vi "FPGAcode4_Test.vi"() -> ()   [LabVIEW 2015]
uses:
  Limits_In.ctl
  Discard_Points.ctl
  Filter_Cluster.ctl
  <vilib>/Platform/TimedLoop/XDataNode/timing_clust.ctl
  <vilib>/Platform/TimedLoop/XDataNode/nitl_modes.ctl
  <vilib>/Platform/TimedLoop/XDataNode/wakeup.ctl
  Detector_Cluster.ctl
  Correlations.ctl
  <vilib>/rvi/Emulation/niFpgaGetClockAttributes.vi
  <vilib>/rvi/Emulation/niFpgaSctlEmulationGetInTimedLoop.vi
  <vilib>/rvi/Emulation/niFpgaEmulationReportErrorSimple.vi
  <vilib>/rvi/Emulation/niFpgaProcessEmulError.vi
  <vilib>/rvi/eio/common/nirviEmuTemplateMethod_errors.vi
  <vilib>/rvi/Emulation/niFpgaCriticalErrorInLSC.vi
  <vilib>/eio/EIONode/EIONode.xnode
  <vilib>/Platform/TimedLoop/XDataNode/XDataNode.xnode
  <vilib>/Platform/TimedLoop/XDataNode/XDNodeRunTimeDep.lvlib
panel:
  in  "User Trigger?":bool
  out "Charge":T1
  out "Mass":T2
  out "Velocity Count":T3
  in  "User Trigger Distance":fxp<+/-,34,18> format="%.3g"
  out "User Trigger":bool
  out "Particles Discarded":i16
  out "All Discard Points":T4
  in  "Boxcar 3 Size Factor":fxp<+/-,32,16>=0.1999969482421875 format="%.2g"
  in  "Charge Error Factor":fxp<+/-,32,16>=1.100006103515625 format="%.2g"
  in  "Max Correlation Factor":fxp<+,32,4>=0.25 format="%.3g"
  in  "Threshold Factor":fxp<+/-,32,16>=1.0 format="%.2g"
  out "DCS 2":bool
  out "Detectors":cluster{"Det 1":i16, "Det 3":i16}
  out "DCS 1":bool
  in  "Limits":T6
  in  "Calibrate":bool=TRUE
  in  "Armed":bool
  out "Plates":bool
  in  "One Shot":bool
  # "These factors above are in the front\npanel so it is possible to experiment\nwith many different configurations\nof the FPGA on the fly. One can even\nchange the relative size of one filter."
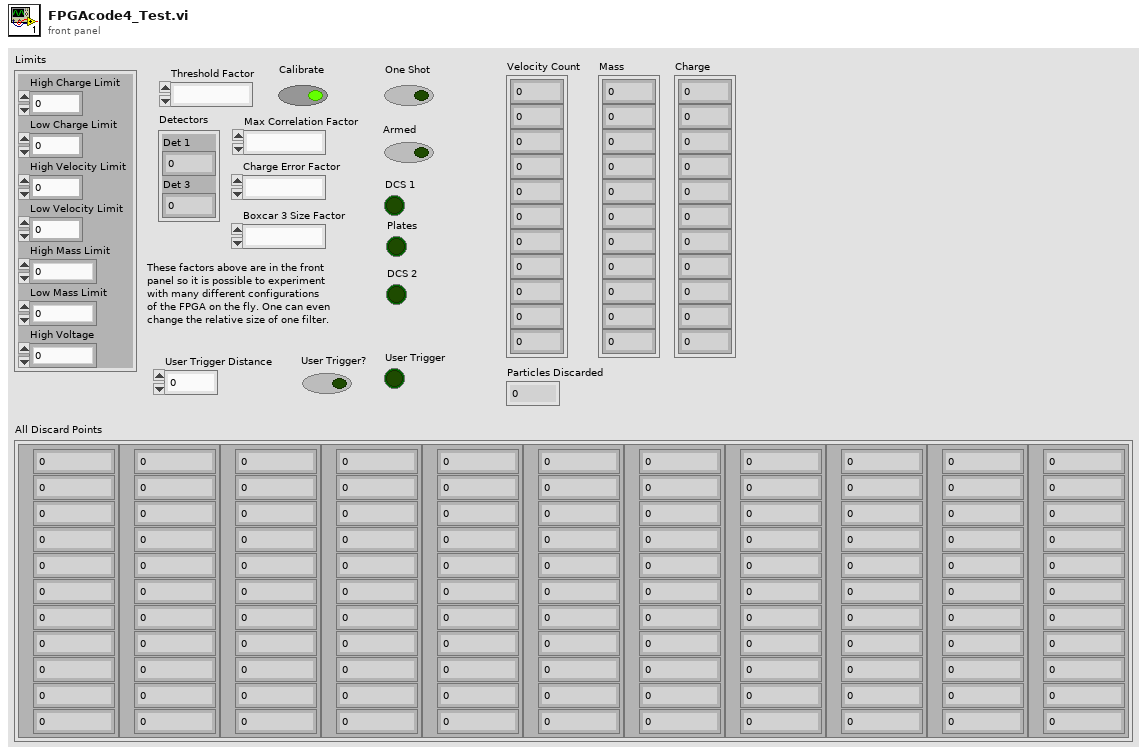
[diagram p1: front panel]
types:
  T1 = cluster{"[0]":fxp<+/-,64,-10>, "[1]":fxp<+/-,64,-10>, "[2]":fxp<+/-,64,-10>, "[3]":fxp<+/-,64,-10>, "[4]":fxp<+/-,64,-10>, "[5]":fxp<+/-,64,-10>, "[6]":fxp<+/-,64,-10>, "[7]":fxp<+/-,64,-10>, "[8]":fxp<+/-,64,-10>, "[9]":fxp<+/-,64,-10>, "[10]":fxp<+/-,64,-10>}
  T2 = cluster{"[0]":fxp<+/-,64,-2>, "[1]":fxp<+/-,64,-2>, "[2]":fxp<+/-,64,-2>, "[3]":fxp<+/-,64,-2>, "[4]":fxp<+/-,64,-2>, "[5]":fxp<+/-,64,-2>, "[6]":fxp<+/-,64,-2>, "[7]":fxp<+/-,64,-2>, "[8]":fxp<+/-,64,-2>, "[9]":fxp<+/-,64,-2>, "[10]":fxp<+/-,64,-2>}
  T3 = cluster{"[0]":i32, "[1]":i32, "[2]":i32, "[3]":i32, "[4]":i32, "[5]":i32, "[6]":i32, "[7]":i32, "[8]":i32, "[9]":i32, "[10]":i32}
  T4 = typedef "Discard_Points.ctl" = cluster{"Discard Points 1":T5, "Discard Points 2":T5, "Discard Points 3":T5, "Discard Points 4":T5, "Discard Points 5":T5, "Discard Points 6":T5, "Discard Points 7":T5, "Discard Points 8":T5, "Discard Points 9":T5, "Discard Points 10":T5, "Discard Points 11":T5}
  T5 = typedef "Filter_Cluster.ctl" = cluster{"1":i32, "2":i32, "3":i32, "4":i32, "5":i32, "6":i32, "7":i32, "8":i32, "9":i32, "10":i32, "11":i32}
  T6 = typedef "Limits_In.ctl" = cluster{"High Charge Limit":fxp<+,32,-41>, "Low Charge Limit":fxp<+,32,-41>, "High Velocity Limit":fxp<+,18,18>, "Low Velocity Limit":fxp<+,18,18>, "High Mass Limit":fxp<+/-,33,-35>, "Low Mass Limit":fxp<+/-,33,-35>, "High Voltage":fxp<+,16,22>}
  T7 = typedef "Detector_Cluster.ctl" = cluster{"Det 1":i32, "Det 2":i32}
  T8 = cluster{"Filter 1":T7, "Filter 2":T7, "Filter 3":T7, "Filter 4":T7}
  T9 = cluster{"Distance to PSU":fxp<+/-,32,5>, "Distance to end of PSU":fxp<+/-,32,5>, "Distance to DCS 2":fxp<+/-,32,5>, "Distance to DCS 1":fxp<+/-,32,5>, "Distance to front of LEIL Chamber":fxp<+/-,32,5>}
  T10 = cluster{"Detector Max Speed Count":i32, "Detector Min Speed Count":i32, "Gap Max Speed Count":i32, "Gap Min Speed Count":i32}
  T11 = cluster{"Distance to PSU":fxp<+/-,64,22>, "Distance to end of PSU":fxp<+/-,64,22>, "Distance to DCS 2":fxp<+/-,64,22>, "Distance to DCS 1":fxp<+/-,64,22>, "Distance to front of LEIL Chamber":fxp<+/-,64,22>}
  T12 = typedef "XDNodeRunTimeDep.lvlib/timing_clust.ctl" = cluster{"Expected End [f-1]":u64, "Actual End [f-1]":u64, "Finished Late? [f-1]":bool, "Expected End [i-1]":u64, "Actual End [i-1]":u64, "Finished Late? [i-1]":bool, "Expected Start [i]":u64, "Actual Start [i]":u64, "Expected Start [f]":u64, "Actual Start [f]":u64, "Source Name":string, "Structure Name":string, "Period":i64, "Deadline":i64, "Offset":i64, "Start":i64, "Priority":i32, "Timeout":i32, "Mode":T13, "Wakeup Reason":T14, "Error":errorcluster, "Source Type":string, "Secondary Source Type":string, "Global End Time":u64, "Global Start Time":u64, "Frame Duration":u64, "Iteration Duration":u64, "Assigned CPU":i32, "I/O Scan Engine Mode":u32}
  T13 = typedef "XDNodeRunTimeDep.lvlib/nitl_modes.ctl" = enum32{"No Change", "Process missed periods, maintain original phase", "Discard missed periods, maintain original phase", "Process missed periods, ignore original phase", "Discard missed periods, ignore original phase"}
  T14 = typedef "XDNodeRunTimeDep.lvlib/wakeup.ctl" = enum32{"Normal", "Aborted", "Asynchronous wakeup", "Timing source error", "Timed loop error", "Timeout"}
  T15 = cluster{"Filter 1":T7, "Filter 2":T7, "Filter 3":T7, "Filter 4":T7}[]
  T16 = cluster{"Distance to PSU":i32, "Distance to end of PSU":i32, "Distance to DCS 2":i32, "Distance to DCS 1":i32, "Distance to front of LEIL Chamber":i32}
  T17 = cluster{"First Detector Count":i32, "Detector Gap Count":i32, "Second Detector Count":i32, "Second Detector Final Count":i32}
  T18 = typedef "Correlations.ctl" = cluster{"First Correlation":i32, "Latest Correlation":i32}
  T19 = cluster{"Detectors":cluster{"Det 1":i16, "Det 3":i16}, cluster{"Det 1":i16, "Det 2":i16}, cluster{"Det 1":i16, "Det 2":i16}, cluster{"Det 1":i16, "Det 2":i16}}
  T20 = cluster{cluster{"Det 1":i16, "Det 2":i16}, cluster{"Det 1":i16, "Det 2":i16}, cluster{"Det 1":i16, "Det 2":i16}, cluster{"Det 1":i16, "Det 2":i16}}
  T21 = cluster{"[0]":u8, "[1]":u8, "[2]":u8, "[3]":u8, "[4]":u8, "[5]":u8, "[6]":u8, "[7]":u8, "[8]":u8, "[9]":u8, "[10]":u8}
  T22 = cluster{"All Discard Points[0]":T5, "All Discard Points[1]":T5, "All Discard Points[2]":T5, "All Discard Points[3]":T5, "All Discard Points[4]":T5, "All Discard Points[5]":T5, "All Discard Points[6]":T5, "All Discard Points[7]":T5, "All Discard Points[8]":T5, "All Discard Points[9]":T5, "All Discard Points[10]":T5}
  T23 = cluster{i32[], fxp<+/-,64,-2>[], fxp<+/-,64,-10>[]}
  T24 = cluster{"IO Module\\AI 0":i16, "IO Module\\AI 1":i16}
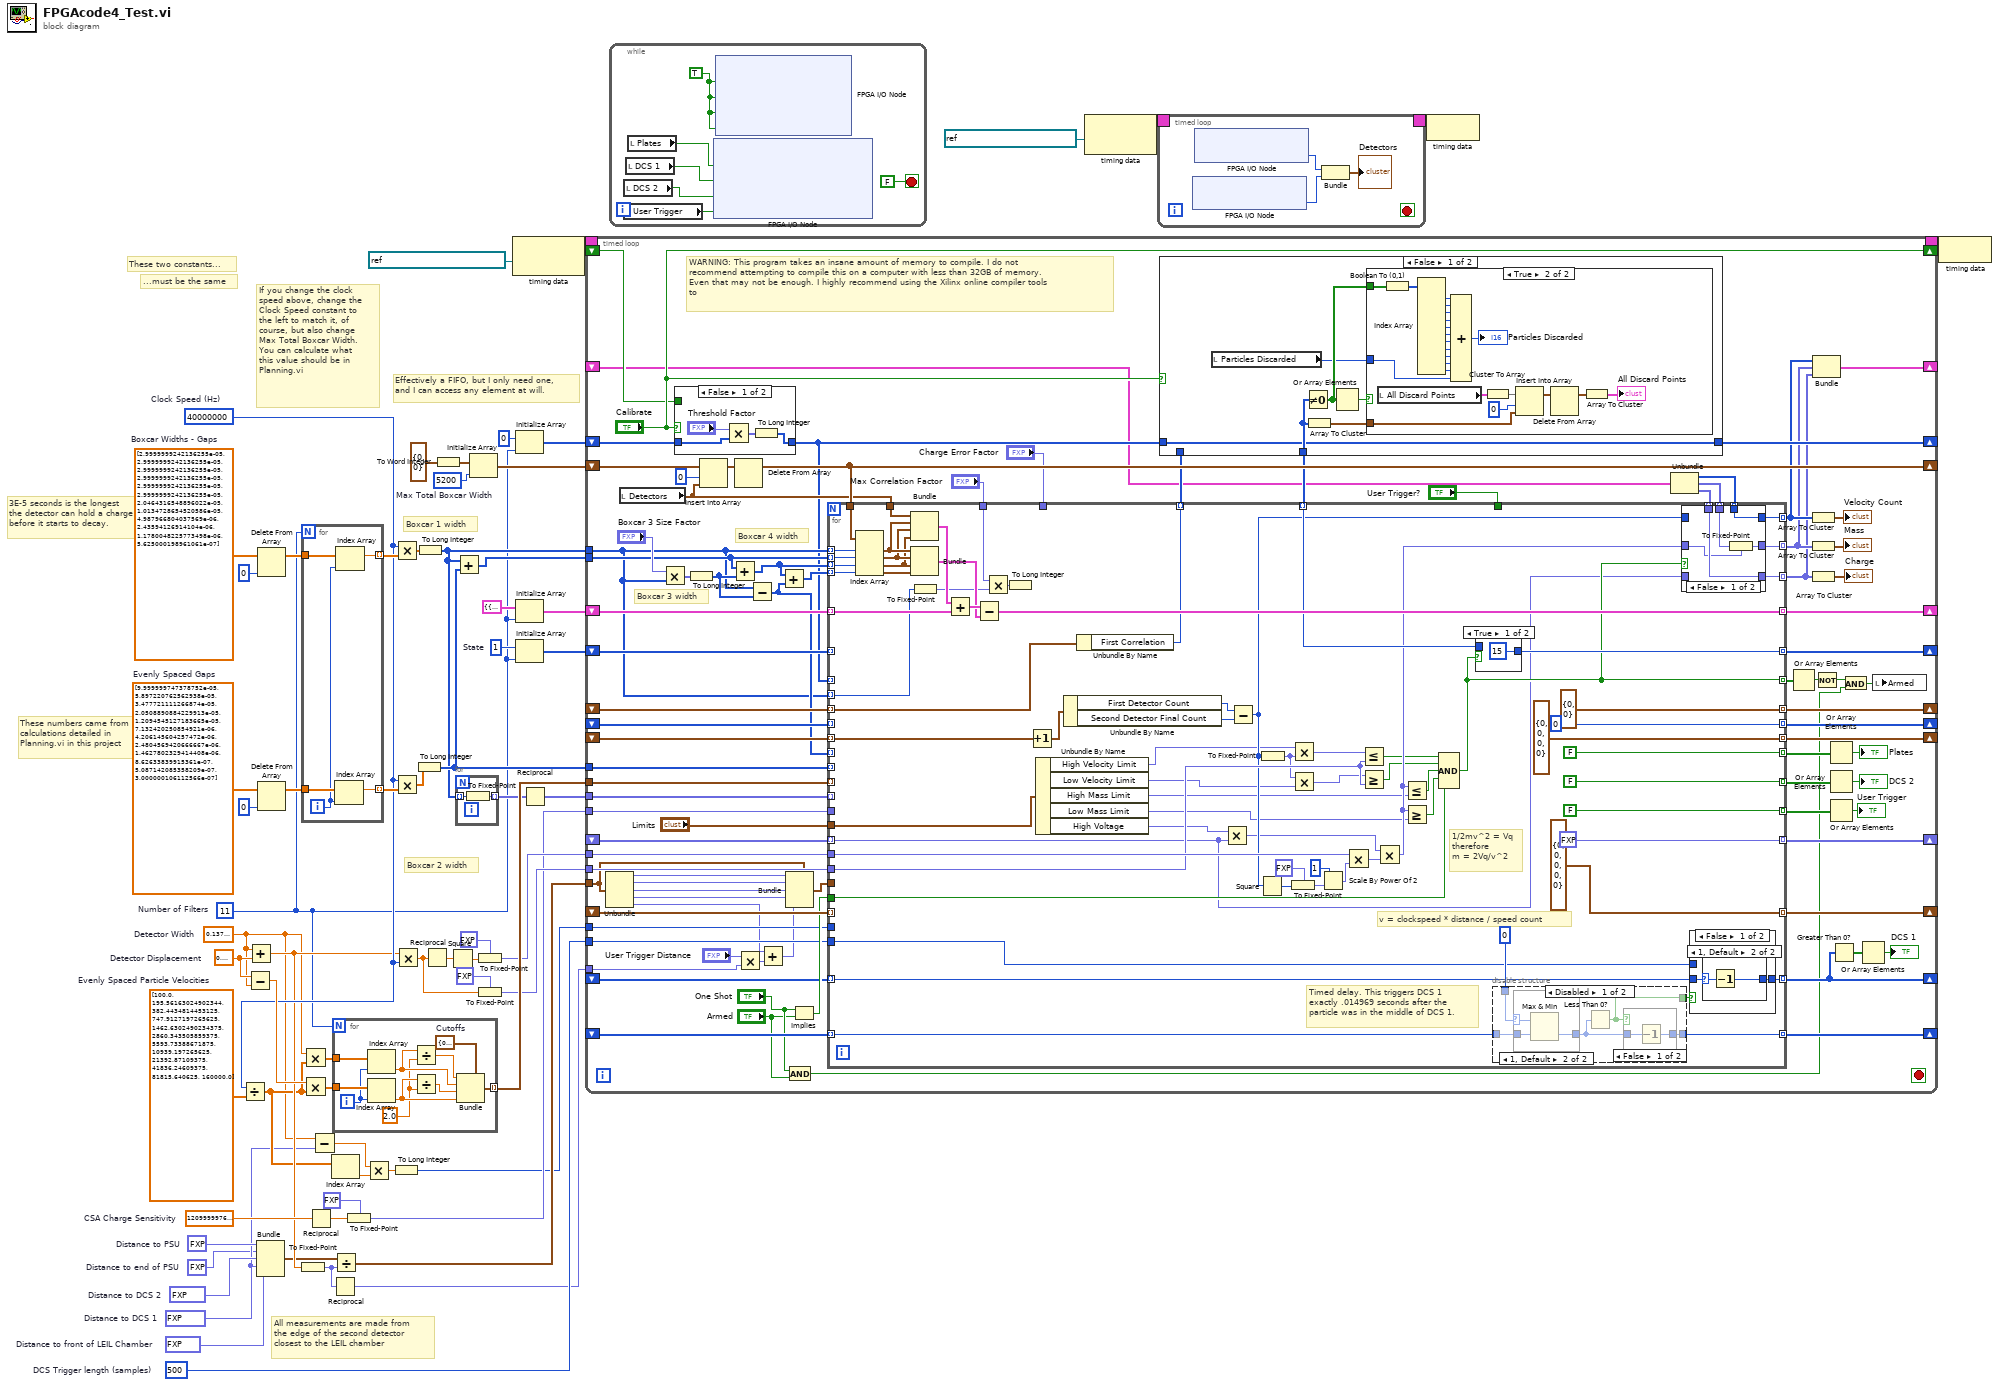
[diagram p0: block diagram]
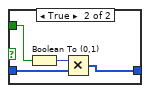
[diagram p2: hidden frame]
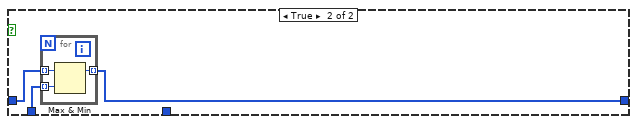
[diagram p4: hidden frame]
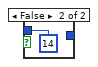
[diagram p5: hidden frame]
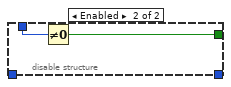
[diagram p11: hidden frame]
diagram:
  w1 = fxp<+/-,32,5> 4.297679997980595  # Distance to front of LEIL Chamber
  w7 = u16 500  # DCS Trigger length (samples)
  w12 = fxp<+/-,32,5> -1.3589000031352043  # Distance to DCS 1
  w16 = fxp<+/-,32,5> 2.6162000000476837  # Distance to DCS 2
  w4 = fxp<+/-,32,5> 1.8999999985098839  # Distance to end of PSU
  w17 = fxp<+/-,32,5> 1.5  # Distance to PSU
  w30 = sgl 12100000000000.0  # CSA Charge Sensitivity
  w52 = u8 1  # State
  w13 = sgl 0.6  # Detector Displacement
  w58 = sgl[] [3e-05, 3e-05, 3e-05, 3e-05, 3e-05, 3e-05, 2.0464317e-05, 1.0134729e-05, 4.987967e-06, 2.4359413e-06, 1.1780048e-06, 5.625e-07]  # Boxcar Widths - Gaps
  w56 = sgl[] [0.0001, 5.8972208e-05, 3.477721e-05, 2.050889e-05, 1.2094545e-05, 7.1324203e-06, 4.2061456e-06, 2.480457e-06, 1.4627802e-06, 8.6263384e-07, 5.087142e-07, 3e-07]  # Evenly Spaced Gaps
  w36 = sgl[] [100.0, 195.56163, 382.44348, 747.9127, 1462.6302, 2860.3435, 5593.734, 10939.197, 21392.871, 41836.246, 81815.64, 160000.0]  # Evenly Spaced Particle Velocities
  w33 = 40000000  # Clock Speed (Hz)
  w8 = sgl 0.138  # Detector Width
  w60 = 5200  # Max Total Boxcar Width
  w5 = 11  # Number of Filters
  # "...must be the same"
  # "These two constants..."
  # "If you change the clock\nspeed above, change the\nClock Speed constant to\nthe left to match it, of\ncourse, but also change\nMax Total Boxcar Width.\nYou can calculate what\nthis value should be in\nPlanning.vi"
  # "All measurements are made from\nthe edge of the second detector\nclosest to the LEIL chamber"
  # "Effectively a FIFO, but I only need one,\nand I can access any element at will."
  # "Boxcar 2 width"
  # "Boxcar 1 width"
  # "3E-5 seconds is the longest\nthe detector can hold a charge\nbefore it starts to decay."
  # "These numbers came from\ncalculations detailed in\nPlanning.vi in this project"
  n1 = Divide(x=w33, y=w36) -> (x/y=w14:sgl[])
  n2 = Subtract(x=w13, y=w8) -> (x-y=w35:sgl)
  n3 = Add(x=w8, y=w13) -> (x+y=w22:sgl)
  n4 = Bundle("Distance to PSU"=w17, "Distance to end of PSU"=w4, "Distance to DCS 2"=w16, "Distance to DCS 1"=w12, "Distance to front of LEIL Chamber"=w1) -> (w21:T9)  [unwired: 1 in]
  n5 = Delete From Array(array=w58, index=0) -> (array with subset deleted=w45:sgl[])  [unwired: 1 in, 1 out]
  n6 = Delete From Array(array=w56, index=0) -> (array with subset deleted=w47:sgl[])  [unwired: 1 in, 1 out]
  n7 = To Fixed-Point(number=w22) -> (fixed-point=w3:fxp<+/-,32,16>)  [unwired: 1 in]
  n8 = for {
    N: w5 -> [_]
    tunnel: w47 -> [w72]
    tunnel: [w69] -> w46 mode=indexing
    tunnel: w45 -> [w71]
    tunnel: [w70] -> w44 mode=indexing
    i -> [w68]
    n9 = Index Array(array=w72, index=w68) -> (element=w69:sgl)
    n10 = Index Array(array=w71, index=w68) -> (element=w70:sgl)
  }
  n11 = Multiply(x=w8, y=w14) -> (x*y=w54:sgl[])
  n12 = Multiply(x=w35, y=w14) -> (x*y=w55:sgl[])
  n13 = Reciprocal(x=w30) -> (1/x=w24:sgl)
  n14 = Subtract(x=w8, y=w12) -> (x-y=w10:sgl)
  n15 = Index Array(array=w14) -> (element=w11:sgl)  [unwired: 1 in]
  n16 = Reciprocal(x=w3) -> (1/x=w2:fxp<+/-,34,18>)
  n17 = for {
    N: w5 -> [_]
    tunnel: w55 -> [w82]
    tunnel: w54 -> [w81]
    tunnel: [w80] -> w49 mode=indexing
    i -> [w79]
    w73 = sgl 2.0 ("y")
    w78 = T10 {"Detector Max Speed Count"=0, "Detector Min Speed Count"=0, "Gap Max Speed Count"=0, "Gap Min Speed Count"=0}  # Cutoffs
    n18 = Index Array(array=w81, index=w79) -> (element=w77:sgl)
    n19 = Index Array(array=w82, index=w79) -> (element=w74:sgl)
    n20 = Divide(x=w77, y=w73) -> (x/y=w76:sgl)
    n21 = Divide(x=w74, y=w73) -> (x/y=w75:sgl)
    n22 = Bundle(cluster=w78, "Detector Max Speed Count"=w76, "Detector Min Speed Count"=w77, "Gap Max Speed Count"=w75, "Gap Min Speed Count"=w74) -> (w80:T10)
  }
  n23 = Divide(x=w21, y=w3) -> (x/y=w20:T11)
  n24 = To Fixed-Point(fixed-point type=fxp<+,32,-43> 0.0, number=w24) -> (fixed-point=w23:fxp<+,32,-43>)
  n25 = Multiply(x=w10, y=w11) -> (x*y=w9:sgl)
  n26 = To Long Integer(number=w9) -> (32bit integer=w6:i32)
  n27 = Multiply(x=w33, y=w44) -> (x*y=w48:sgl[])
  n28 = Multiply(x=w33, y=w46) -> (x*y=w53:sgl[])
  n29 = Multiply(x=w22, y=w33) -> (x*y=w27:sgl)
  n30 = To Long Integer(number=w53) -> (32bit integer=w43:i32[])
  n31 = To Long Integer(number=w48) -> (32bit integer=w39:i32[])
  n32 = Reciprocal(x=w27) -> (1/x=w32:sgl)
  n33 = To Word Integer(number=T7 {"Det 1"=0, "Det 2"=0} ("Detectors")) -> (16bit integer=w42:cluster{"Det 1":i16, "Det 2":i16})
  n34 = Square(x=w32) -> (x^2=w31:sgl)
  n35 = Add(x=w39, y=w43) -> (x+y=w15:i32[])
  n36 = for {
    tunnel: w39 -> [w84] mode=indexing
    tunnel: [w83] -> w38 mode=indexing
    n37 = To Fixed-Point(number=w84) -> (fixed-point=w83:fxp<+/-,32,32>)  [unwired: 1 in]
  }
  n38 = Initialize Array(w42, w60) -> (w61:cluster{"Det 1":i16, "Det 2":i16}[])
  n39 = To Fixed-Point(fixed-point type=fxp<+/-,32,-45> 0.0, number=w31) -> (fixed-point=w34:fxp<+/-,32,-45>)
  n40 = To Fixed-Point(fixed-point type=fxp<+,32,32> 0.0, number=w27) -> (fixed-point=w25:fxp<+,32,32>)
  n41 = node-c288(refnum<k21> "40 MHz Onboard Clock" ("Source Name")) -> (w64:T12)
  n42 = Initialize Array(0 ("element"), w5) -> (w18:i32[])
  n43 = Initialize Array(T8 {"Filter 1"={"Det 1"=0, "Det 2"=0}, "Filter 2"={"Det 1"=0, "Det 2"=0}, "Filter 3"={"Det 1"=0, "Det 2"=0}, "Filter 4"={"Det 1"=0, "Det 2"=0}} ("cluster"), w5) -> (w50:T15)
  n44 = Initialize Array(w52, w5) -> (w51:u8[])
  n45 = Reciprocal(x=w38) -> (1/x=w37:fxp<+/-,34,2>[])
  n46 = timed-loop {
    timing: w64 -> [_]
    timing-out: [_] -> w63
    shift-right: [w169] -> _
    shift-left: w61 -> [w172]
    shift-right: [w168] -> _
    shift-left: w50 -> [w161]
    shift-right: [w166] -> _
    shift-left: w51 -> [w167]
    shift-right: [w165] -> _
    shift-left: _ -> [w164]
    shift-right: [w163] -> _
    shift-left: _ -> [w162]
    tunnel: w49 -> [w159]
    shift-right: [w158] -> _
    shift-left: _ -> [w157]
    tunnel: w39 -> [w146]
    tunnel: w15 -> [w152]
    tunnel: w43 -> [w147]
    tunnel: w37 -> [w145]
    shift-right: [w143] -> _
    shift-left: _ -> [w142]
    tunnel: w34 -> [w141]
    tunnel: w23 -> [w140]
    tunnel: w25 -> [w139]
    tunnel: w20 -> [w117]
    shift-right: [w138] -> _
    shift-left: _ -> [w137]
    shift-right: [w135] -> _
    shift-left: w18 -> [w133]
    shift-right: ["Calibrate"] -> _
    shift-left: _ -> [w130]
    tunnel: w7 -> [w128]
    tunnel: w6 -> [w127]
    shift-right: [w124] -> _
    shift-left: _ -> [w126]
    shift-right: [w122] -> _
    shift-left: _ -> [w121]
    tunnel: w2 -> [w120]
    shift-right: [w91] -> _
    shift-left: _ -> [w90]
    stop <- _ stop-if-true
    # "WARNING: This program takes an insane amount of memory to compile. I do not\nrecommend attempting to compile this on a computer with less than 32GB of memory.\nEven that may not be enough. I highly recommend using the Xilinx online compiler tools\nto"
    # "Boxcar 3 width"
    # "Boxcar 4 width"
    n47 = Unbundle(w117) -> ("Distance to PSU"=w118:fxp<+/-,64,22>, "Distance to end of PSU"=w116:fxp<+/-,64,22>, "Distance to DCS 2"=w115:fxp<+/-,64,22>, "Distance to DCS 1"=w112:fxp<+/-,64,22>, "Distance to front of LEIL Chamber"=w111:fxp<+/-,64,22>)
    n48 = local read "Detectors"() -> (w160:cluster{"Det 1":i16, "Det 3":i16})
    n49 = Multiply(x="Boxcar 3 Size Factor", y=w146) -> (x*y=w154:fxp<+/-,64,48>[])
    n50 = case shown="False" "Calibrate" {
      tunnel: w133 -> [w174 w180]
      tunnel: [w173 w178] -> w132
      tunnel: w130 -> [_ w179]
      frame False {
        n51 = Multiply(x="Threshold Factor", y=w174) -> (x*y=w175:fxp<+/-,64,48>[])
        n52 = To Long Integer(number=w175) -> (32bit integer=w173:i32[])
      }
      frame True {
        n53 = Boolean To (0,1)(Boolean=w179) -> (0, 1=w177:i16)
        n54 = Multiply(x=w177, y=w180) -> (x*y=w178:i32[])
      }
    }
    n55 = To Long Integer(number=w154) -> (32bit integer=w155:i32[])
    n56 = Insert Into Array(array=w172, index=0, new element=w160) -> (w171:cluster{"Det 1":i16, "Det 2":i16}[])
    n57 = Add(x=w152, y=w155) -> (x+y=w151:i32[])
    n58 = Delete From Array(array=w171) -> (array with subset deleted=w169:cluster{"Det 1":i16, "Det 2":i16}[])  [unwired: 2 in, 1 out]
    n59 = Multiply(x="User Trigger Distance", y=w120) -> (x*y=w113:fxp<+/-,64,34>)
    n60 = Subtract(x=w146, y=w155) -> (x-y=w149:i32[])
    n61 = Add(x=w111, y=w113) -> (x+y=w110:fxp<+/-,64,35>)
    n62 = Add(x=w151, y=w149) -> (x+y=w150:i32[])
    n63 = Bundle(cluster=w117, "Distance to PSU"=w118, "Distance to end of PSU"=w116, "Distance to DCS 2"=w115, "Distance to DCS 1"=w112, "Distance to front of LEIL Chamber"=w110) -> (w114:T11)
    n64 = And(x="One Shot", y="Armed") -> (x .and. y?=w100:bool)
    n65 = Implies(1:"Armed", 2:"One Shot") -> (0:w129:bool)
    n66 = Unbundle(w90) -> (w89:i32[], w88:fxp<+/-,64,-2>[], w87:fxp<+/-,64,-10>[])
    n67 = for {
      tunnel: w169 -> [w289]
      tunnel: [w275] -> w168 mode=indexing
      tunnel: w167 -> [_] mode=indexing
      tunnel: [w288] -> w166 mode=indexing
      tunnel: w132 -> [_] mode=indexing
      tunnel: [T18 {"First Correlation"=0, "Latest Correlation"=0} ("input cluster")] -> w165 mode=indexing
      tunnel: w164 -> [w286] mode=indexing
      tunnel: [0] -> w163 mode=indexing
      tunnel: w162 -> [_] mode=indexing
      tunnel: w161 -> [w279] mode=indexing
      tunnel: w160 -> [w284]
      tunnel: w159 -> [_] mode=indexing
      tunnel: [T17 {"First Detector Count"=0, "Detector Gap Count"=0, "Second Detector Count"=0, "Second Detector Final Count"=0} ("Cutoffs")] -> w158 mode=indexing
      tunnel: w157 -> [w273] mode=indexing
      tunnel: w146 -> [w272] mode=indexing
      tunnel: w152 -> [w271] mode=indexing
      tunnel: w151 -> [w270] mode=indexing
      tunnel: w150 -> [w269] mode=indexing
      tunnel: w146 -> [w238] mode=indexing
      tunnel: "Max Correlation Factor" -> [w268]
      tunnel: w149 -> [_] mode=indexing
      tunnel: w147 -> [_] mode=indexing
      tunnel: "Charge Error Factor" -> [_]
      tunnel: [w267] -> w136 mode=indexing
      tunnel: w145 -> [_] mode=indexing
      tunnel: "Limits" -> [w266]
      tunnel: [fxp<+/-,64,-10> 0.0] -> w143 mode=indexing
      tunnel: w142 -> [w247] mode=indexing
      tunnel: w141 -> [w264]
      tunnel: w140 -> [_]
      tunnel: w139 -> [w263]
      tunnel: w114 -> [_]
      tunnel: [T16 {"Distance to PSU"=0, "Distance to end of PSU"=0, "Distance to DCS 2"=0, "Distance to DCS 1"=0, "Distance to front of LEIL Chamber"=0}] -> w138 mode=indexing
      tunnel: w137 -> [_] mode=indexing
      tunnel: [w261] -> w134 mode=indexing
      tunnel: w129 -> [w260]
      tunnel: w128 -> [w258]
      tunnel: w127 -> [_]
      tunnel: [w257] -> w124 mode=indexing
      tunnel: w126 -> [w256] mode=indexing
      tunnel: [w254] -> w122 mode=indexing
      tunnel: w121 -> [w253] mode=indexing
      tunnel: [FALSE] -> w109 mode=indexing
      tunnel: [FALSE] -> w107 mode=indexing
      tunnel: [FALSE] -> w106 mode=indexing
      tunnel: [w249] -> w103 mode=indexing
      tunnel: [w243] -> w94 mode=indexing
      tunnel: [w248] -> w92 mode=indexing
      tunnel: [w246] -> w93 mode=indexing
      tunnel: w89 -> [w242] mode=indexing
      tunnel: w88 -> [w241] mode=indexing
      tunnel: w87 -> [w240] mode=indexing
      tunnel: "User Trigger?" -> [_]
      # "v = clockspeed * distance / speed count"
      # "1/2mv^2 = Vq\ntherefore\nm = 2Vq/v^2"
      # "Timed delay. This triggers DCS 1\nexactly .014969 seconds after the\nparticle was in the middle of DCS 1."
      n68 = Index Array(array=w289, index #1=w272, index #2=w271, index #3=w270, index #4=w269) -> (element #1=w282:cluster{"Det 1":i16, "Det 2":i16}, element #2=w281:cluster{"Det 1":i16, "Det 2":i16}, element #3=w280:cluster{"Det 1":i16, "Det 2":i16}, element #4=w283:cluster{"Det 1":i16, "Det 2":i16})
      n69 = Bundle("Detectors"=w284, w282, w281, w280) -> (w278:T19)  [unwired: 1 in]
      n70 = Bundle(w282, w281, w280, w283) -> (w276:T20)  [unwired: 1 in]
      n71 = To Fixed-Point(number=w238) -> (fixed-point=w237:fxp<+/-,32,32>)  [unwired: 1 in]
      n72 = Add(x=w278, y=w279) -> (x+y=w277:T8)
      n73 = Subtract(x=w277, y=w276) -> (x-y=w275:T8)
      n74 = Multiply(x=w268, y=w237) -> (x*y=w239:fxp<+/-,64,36>)
      n75 = To Long Integer(number=w239) -> ()  [unwired: 1 out]
      n76 = Increment(x=w273) -> (x+1=w236:T17)
      n77 = Unbundle By Name(w266) -> ("High Velocity Limit"=w218:fxp<+,18,18>, "Low Velocity Limit"=w219:fxp<+,18,18>, "High Mass Limit"=w227:fxp<+/-,33,-35>, "Low Mass Limit"=w228:fxp<+/-,33,-35>, "High Voltage"=w222:fxp<+,16,22>)
      n78 = Unbundle By Name(w236) -> ("First Detector Count"=w235:i32, "Second Detector Final Count"=w234:i32)
      n79 = Unbundle By Name(w286) -> ("First Correlation"=w261:i32)
      n80 = Multiply(x=w222, y=w247) -> (x*y=w229:fxp<+/-,64,12>)
      n81 = Subtract(x=w235, y=w234) -> (x-y=w244:i32)
      n82 = Square(x=w244) -> (x^2=w233:i32)
      n83 = To Fixed-Point(number=w244) -> (fixed-point=w217:fxp<+/-,32,32>)  [unwired: 1 in]
      n84 = To Fixed-Point(fixed-point type=fxp<+,32,32> 0.0, number=w233) -> (fixed-point=w231:fxp<+,32,32>)
      n85 = Multiply(x=w218, y=w217) -> (x*y=w216:fxp<+/-,50,50>)
      n86 = Multiply(x=w217, y=w219) -> (x*y=w215:fxp<+/-,50,50>)
      n87 = Scale By Power Of 2(n=i16 1, x=w231) -> (x*2^n=w221:fxp<+,32,32>)
      n88 = Multiply(x=w264, y=w221) -> (x*y=w230:fxp<+/-,64,-13>)
      n89 = Less Or Equal?(x=w216, y=w263) -> (x <= y?=w226:bool)
      n90 = Greater Or Equal?(x=w215, y=w263) -> (x >= y?=w225:bool)
      n91 = Multiply(x=w229, y=w230) -> (x*y=w245:fxp<+/-,64,-2>)
      n92 = Less Or Equal?(x=w245, y=w227) -> (x <= y?=w224:bool)
      n93 = Greater Or Equal?(x=w245, y=w228) -> (x >= y?=w223:bool)
      n94 = Compound Arithmetic op=AND(w226, w225, w224, w223, w260) -> (w249:bool)
      n95 = case shown="True" w249 {
        tunnel: [u8 15 ("Det 3") _] -> w288
        tunnel: [_ u8 14 ("Det 3")] -> w267
        frame True {
        }
        frame False {
        }
      }
      n96 = disable-structure shown="Disabled" {
        disable-tunnel: 0 -> [w310 w318]
        disable-tunnel: [w306 w317] -> w255
        disable-tunnel: [w308 _] -> w254
        disable-tunnel: w253 -> [w309 _]
        frame Disabled {
          n97 = case shown="1, Default" w310 {
            selector: w310 -> [_ w316]
            tunnel: [w313 w314] -> w307
            tunnel: w309 -> [w313 w315]
            frame 0 {
            }
            frame 1, Default {
              n98 = Max & Min(x=w316, y=w315) -> (min(x,y)=w314:i32)  [unwired: 1 out]
            }
          }
          n99 = Less Than 0?(x=w307) -> (x < 0?=w306:bool)
          n100 = case shown="False" w306 {
            tunnel: w307 -> [w312 _]
            tunnel: [w311 _] -> w308
            frame False {
              n101 = Decrement(x=w312) -> (x-1=w311:i32)
            }
            frame True {
            }
          }
        }
        frame Enabled {
          n102 = Not Equal To 0?(x=w318) -> (x != 0?=w317:bool)
        }
      }
      n103 = case shown="False" w249 {
        tunnel: [w295 w299] -> w248
        tunnel: w247 -> [_ w299]
        tunnel: [w293 w297] -> w246
        tunnel: w245 -> [w292 w297]
        tunnel: w244 -> [_ w298]
        tunnel: [w296 w298] -> w243
        tunnel: w242 -> [w296 _]
        tunnel: w241 -> [w294 _]
        tunnel: w240 -> [w295 _]
        frame False {
          n104 = To Fixed-Point(fixed-point type=w292, number=w294) -> (fixed-point=w293:fxp<+/-,64,-2>)
        }
        frame True {
        }
      }
      n105 = case shown="False" w255 {
        tunnel: w258 -> [_ w305]
        tunnel: [w300 w305] -> w257
        tunnel: w256 -> [w301 _]
        frame False {
          n106 = case shown="1, Default" w301 {
            selector: w301 -> [w302 w304]
            tunnel: [w302 w303] -> w300
            frame 0 {
            }
            frame 1, Default {
              n107 = Decrement(x=w304) -> (x-1=w303:u16)
            }
          }
        }
        frame True {
        }
      }
    }
    n108 = case shown="False" "Calibrate" {
      tunnel: w136 -> [w185 _]
      tunnel: w132 -> [w181 w211]
      tunnel: [w181 w209] -> w135
      tunnel: w134 -> [_ w210]
      frame False {
        n109 = local read "Particles Discarded"() -> (w183:i16)
        n110 = Not Equal To 0?(x=w185) -> (x != 0?=w184:bool[])
        n111 = Array To Cluster(array=w185) -> (cluster=w186:T21)
        n112 = Or Array Elements(Boolean array=w184) -> (logical OR=w182:bool)
        n113 = case shown="True" w182 {
          tunnel: w186 -> [_ w202]
          tunnel: w184 -> [_ w188]
          tunnel: w183 -> [_ w187]
          frame False {
          }
          frame True {
            n114 = local read "All Discard Points"() -> (w208:T4)
            n115 = Boolean To (0,1)(Boolean=w188) -> (0, 1=w189:i16[])
            n116 = Index Array(array=w189) -> (element #1=w191:i16, element #2=w192:i16, element #3=w193:i16, element #4=w194:i16, element #5=w195:i16, element #6=w196:i16, element #7=w197:i16, element #8=w198:i16, element #9=w199:i16, element #10=w200:i16, element #11=w190:i16)  [unwired: 11 in]
            n117 = Compound Arithmetic op=ADD(w191, w192, w193, w194, w195, w196, w197, w198, w199, w200, w190, w187) -> (→"Particles Discarded":i16)
            n118 = Cluster To Array(cluster=w208) -> (array=w204:T5[])
            n119 = Insert Into Array(array=w204, index=0, new element=w202) -> (w206:T5[])
            n120 = Delete From Array(array=w206) -> (array with subset deleted=w203:T5[])  [unwired: 2 in, 1 out]
            n121 = Array To Cluster(array=w203) -> (cluster=→"All Discard Points":T22)
          }
        }
      }
      frame True {
        n122 = for {
          tunnel: w210 -> [w214] mode=indexing
          tunnel: w211 -> [w213] mode=indexing
          tunnel: [w212] -> w209 mode=indexing
          n123 = Max & Min(x=w213, y=w214) -> (max(x,y)=w212:i32)  [unwired: 1 out]
        }
      }
    }
    n124 = Or Array Elements(Boolean array=w103) -> (logical OR=w97:bool)
    n125 = Array To Cluster(array=w94) -> (cluster=→"Velocity Count":T3)
    n126 = Array To Cluster(array=w93) -> (cluster=→"Mass":T2)
    n127 = Array To Cluster(array=w92) -> (cluster=→"Charge":T1)
    n128 = Bundle(w94, w93, w92) -> (w91:T23)  [unwired: 1 in]
    n129 = Not(x=w97) -> (.not. x?=w102:bool)
    n130 = Or Array Elements(Boolean array=w109) -> (logical OR=→"Plates":bool)
    n131 = Or Array Elements(Boolean array=w107) -> (logical OR=→"DCS 2":bool)
    n132 = Or Array Elements(Boolean array=w106) -> (logical OR=→"User Trigger":bool)
    n133 = Greater Than 0?(x=w124) -> (x > 0?=w123:bool[])
    n134 = And(x=w102, y=w100) -> (x .and. y?=w101:bool)
    n135 = Or Array Elements(Boolean array=w123) -> (logical OR=→"DCS 1":bool)
    n136 = local write "Armed"(w101) -> ()
  }
  n137 = while {
    stop <- FALSE stop-if-true
    w322 = TRUE ("IO Module\\PFI Enable")
    n138 = local read "DCS 2"() -> (w323:bool)
    n139 = local read "User Trigger"() -> (w321:bool)
    n140 = local read "DCS 1"() -> (w324:bool)
    n141 = local read "Plates"() -> (w325:bool)
    n142 = xnode "FPGA I/O Node"("IO Module\\PFI 0 Wr Data"=w325, "IO Module\\PFI 1 Wr Data"=w324, "IO Module\\PFI 2 Wr Data"=w323, "IO Module\\PFI 3 Wr Data"=w321) -> ()  [unwired: 4 in, 4 out]
    n143 = xnode "FPGA I/O Node"("IO Module\\PFI 0 WE"=w322, "IO Module\\PFI 1 WE"=w322, "IO Module\\PFI 2 WE"=w322, "IO Module\\PFI 3 WE"=w322) -> ()  [unwired: 4 in, 4 out]
  }
  n144 = node-c288(refnum<k21> "IO Module\\Data Clock" ("Source Name")) -> (w67:T12)
  n145 = timed-loop {
    timing: w67 -> [_]
    timing-out: [_] -> w66
    stop <- _ stop-if-true
    n146 = xnode "FPGA I/O Node"() -> ("IO Module\\AI 1"=w328:i16)  [unwired: 1 in, 1 out]
    n147 = xnode "FPGA I/O Node"() -> ("IO Module\\AI 0"=w329:i16)  [unwired: 1 in, 1 out]
    n148 = Bundle("IO Module\\AI 0"=w329, "IO Module\\AI 1"=w328) -> (→"Detectors":T24)  [unwired: 1 in]
  }
  n149 = node-c288(w66) -> ()
  n150 = node-c288(w63) -> ()
